vi "initialOptions.vi"(9 "index":cluster{"row":i32, "column":i32}, 10 "State in":cluster{"Value":i32, "Options":i32[]}[][](array[cluster])) -> (2 "State out":cluster{"Value":i32, "Options":i32[]}[][](array[cluster]))   [LabVIEW 2014, in "SudokuState.lvclass"]
uses:
  <userlib>/AdvancedDataStructures/ClassBased/Applications/SudukuSolver/SudukuState/SudokuState.lvclass
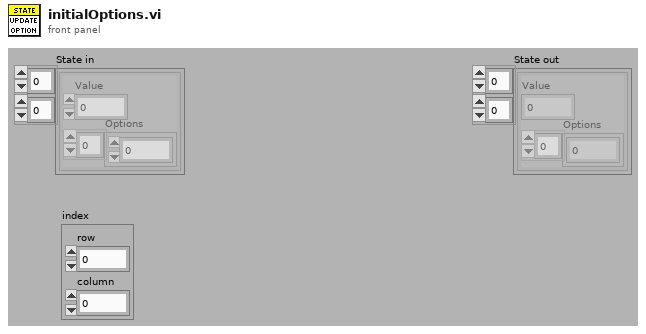
[diagram p1: front panel]
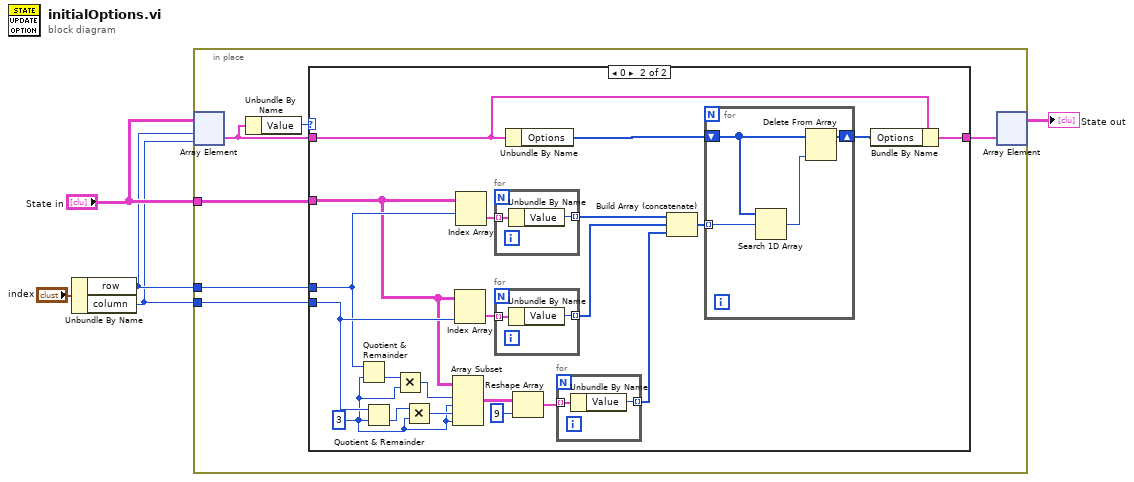
[diagram p0: block diagram]
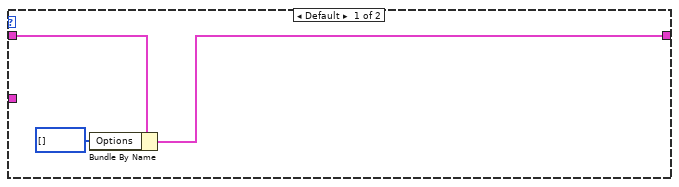
[diagram p2: hidden frame]
diagram:
  n1 = Unbundle By Name("index") -> ("row"=w2:i32, "column"=w1:i32)
  n2 = in-place {
    in-place-border: "State in" -> [w8]
    in-place-border: w2 -> [w7]
    in-place-border: w1 -> [w6]
    n3 = in-place-array #1("State in", w2, w1) -> (w10:cluster{"Value":i32, "Options":i32[]})
    n4 = Unbundle By Name(w10) -> ("Value"=w11:i32)
    n5 = case shown="0" w11 {
      tunnel: w10 -> [w14 w29]
      tunnel: [w12 w27] -> w9
      tunnel: w8 -> [_ w24]
      tunnel: w7 -> [_ w25]
      tunnel: w6 -> [_ w26]
      frame Default {
        n6 = Bundle By Name(cluster=w14, "Options"=i32[] []) -> (w12:cluster{"Value":i32, "Options":i32[]})
      }
      frame 0 {
        w21 = 3 ("y")
        n7 = Quotient & Remainder(x=w25, y=w21) -> (floor(x/y)=w16:i32)  [unwired: 1 out]
        n8 = Quotient & Remainder(x=w26, y=w21) -> (floor(x/y)=w15:i32)  [unwired: 1 out]
        n9 = Multiply(x=w16, y=w21) -> (x*y=w23:i32)
        n10 = Multiply(x=w15, y=w21) -> (x*y=w22:i32)
        n11 = Array Subset(array=w24, index (row)=w23, length (row)=w21, index (col)=w22, length (col)=w21) -> (w20:cluster{"Value":i32, "Options":i32[]}[][])
        n12 = Index Array(array=w24, index (col)=w26) -> (element=w34:cluster{"Value":i32, "Options":i32[]}[])  [unwired: 1 in]
        n13 = Index Array(array=w24, index (row)=w25) -> (element=w35:cluster{"Value":i32, "Options":i32[]}[])  [unwired: 1 in]
        n14 = for {
          tunnel: w35 -> [w45] mode=indexing
          tunnel: [w44] -> w32 mode=indexing
          n15 = Unbundle By Name(w45) -> ("Value"=w44:i32)
        }
        n16 = for {
          tunnel: w34 -> [w43] mode=indexing
          tunnel: [w42] -> w33 mode=indexing
          n17 = Unbundle By Name(w43) -> ("Value"=w42:i32)
        }
        n18 = Unbundle By Name(w29) -> ("Options"=w30:i32[])
        n19 = Reshape Array(w20, 9 ("dimension size")) -> (w18:cluster{"Value":i32, "Options":i32[]}[])
        n20 = for {
          tunnel: w18 -> [w37] mode=indexing
          tunnel: [w36] -> w17 mode=indexing
          n21 = Unbundle By Name(w37) -> ("Value"=w36:i32)
        }
        n22 = Build Array (concatenate)(w32, w33, w17) -> (w31:i32[])
        n23 = for {
          tunnel: w31 -> [w41] mode=indexing
          shift-right: [w38] -> w28
          shift-left: w30 -> [w40]
          n24 = Search 1D Array(1D array=w40, element=w41) -> (index of element=w39:i32)  [unwired: 1 in]
          n25 = Delete From Array(array=w40, index=w39) -> (array with subset deleted=w38:i32[])  [unwired: 1 in, 1 out]
        }
        n26 = Bundle By Name(cluster=w29, "Options"=w28) -> (w27:cluster{"Value":i32, "Options":i32[]})
      }
    }
    n27 = in-place-array #1(w9) -> (→"State out":cluster{"Value":i32, "Options":i32[]}[][])  [unwired: 2 out]
  }
